vi "LinxI2cWrite.vi"(5 "EOF":u8, 7 "I2C Channel":u8, 8 "Error In":errorcluster, 9 "Data":u8[](array[numeric]), 10 "Slave Address":u8, 11 "LINX Resource":T1) -> (0 "Error Out":errorcluster, 3 "LINX Resource":T1)   [LabVIEW 2019, in "LMH-LINX.lvlib" / "Local IO.lvlib"]
uses:
  <vilib>/MakerHub/LINX/Private/Local IO/Local IO.lvlib
  <vilib>/MakerHub/LINX/Private/Type Defs/LINX Ref.ctl
  <vilib>/MakerHub/LINX/Private/Type Defs/Platform.ctl
  <vilib>/MakerHub/LINX/Private/Type Defs/Interface.ctl
  <vilib>/MakerHub/LINX/Private/Device/Type Defs/LINX Device Config.ctl
  <vilib>/MakerHub/LINX/Private/Device/Type Defs/TCP Config.ctl
  <vilib>/MakerHub/LINX/Private/Device/Type Defs/Channels.ctl
  <vilib>/MakerHub/LINX/Resources/liblinxdevice.dll
  <vilib>/MakerHub/LINX/LMH-LINX.lvlib
  <vilib>/MakerHub/LINX/Private/Device/Device.lvlib
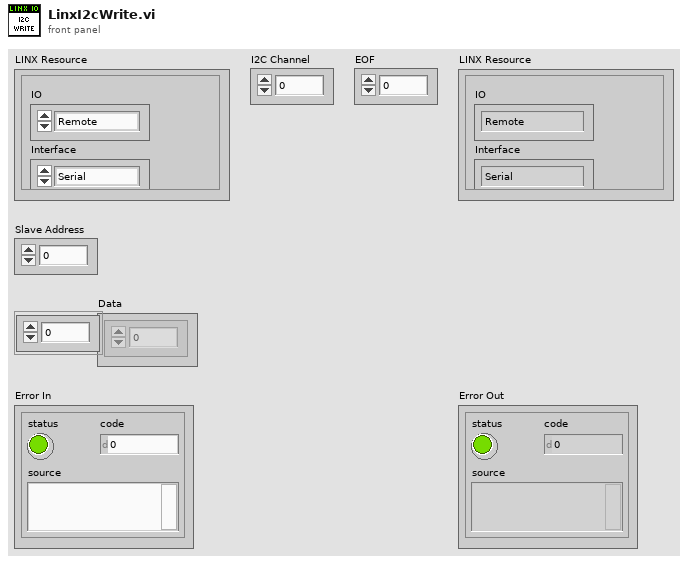
[diagram p1: front panel]
types:
  T1 = typedef "LMH-LINX.lvlib/LINX Ref.ctl" = cluster{"IO":T2, "Interface":T3, "LINX Device Config":T4}
  T2 = typedef "LMH-LINX.lvlib/Platform.ctl" = enum16{"Remote", "Local"}
  T3 = typedef "LMH-LINX.lvlib/Interface.ctl" = enum16{"Serial", "TCP"}
  T4 = typedef "LMH-LINX.lvlib/Device.lvlib/LINX Device Config.ctl" = cluster{"Interface":T3, "COM Port":refnum<visa-resource-name>, "TCP Configuration":T5, "Device Family":u8, "Device ID":u8, "Device Name":string, "TCP Ref":refnum<k5>, "Channels":T6}
  T5 = typedef "LMH-LINX.lvlib/Device.lvlib/TCP Config.ctl" = cluster{"IP Address":string, "Port":u16}
  T6 = typedef "LMH-LINX.lvlib/Channels.ctl" = cluster{"DI":u8[], "DO":u8[], "AI":u8[], "AO":u8[], "PWM":u8[], "QE":u8[], "UART":u8[], "I2C 2":u8[], "SPI":u8[], "CAN":u8[], "Servo":u8[], "AI Ref (V)":dbl, "AI Resolution (Bits)":u8, "AO Ref (V)":dbl, "AO Resolution (Bits)":u8}
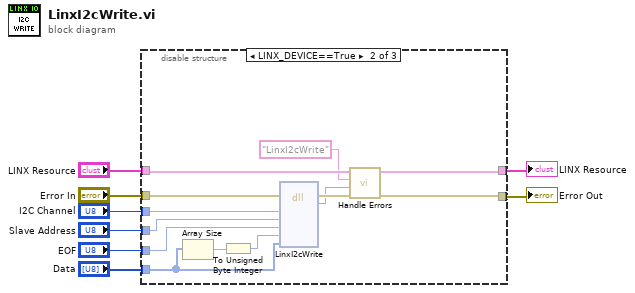
[diagram p0: block diagram]
diagram:
  n1 = disable-structure shown="LINX_DEVICE==True" {
    disable-tunnel: "LINX Resource" -> [w10 w22 w24]
    disable-tunnel: "Error In" -> [w9 w23 w25]
    disable-tunnel: [w9 w20 w25] -> w6
    disable-tunnel: [w10 w21 w24] -> w5
    disable-tunnel: "I2C Channel" -> [_ w16 _]
    disable-tunnel: "Slave Address" -> [_ w15 _]
    disable-tunnel: "EOF" -> [_ w14 _]
    disable-tunnel: "Data" -> [_ w13 _]
    frame condition #0 (active) {
    }
    frame condition #1 {
      n2 = Array Size(array=w13) -> (size(s)=w12:i32)
      n3 = To Unsigned Byte Integer(number=w12) -> (unsigned 8bit integer=w11:u8)
      n4 = dll-call lib="E:/lv2019/dist/vi.lib/MakerHub/LINX/Resources/liblinxdevice.*" fn="LinxI2cWrite"(error in=w23, "channel"=w16, "slaveAddress"=w15, "eofConfig"=w14, "numBytes"=w11, "sendBuffer"=w13) -> (error out=w19:errorcluster, "LinxStatus"=w18:i32)  [unwired: 7 in, 1 out]
      n5 = call <vilib>:"Handle Errors.vi"("Error In"=w19, "LinxStatus"=w18, "Function Name"="LinxI2cWrite", "LINX Resource"=w22) -> ("Error Out"=w20:errorcluster, "LINX Resource"=w21:T1)  [unwired: 6 in]
    }
    frame condition #2 {
      # "myRIO Support Disabled"
    }
  }
  "Error Out" <- w6
  "LINX Resource" <- w5
